vi "Zig Zag Global.vi"() -> ()   [LabVIEW 2017]
panel:
  in  "Need New Zig Zag Values":bool=TRUE
  in  "Zig Zag Finished":bool
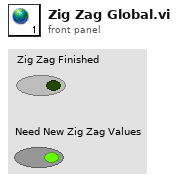
[diagram p1: front panel]
diagram:
